vi "#ch_choose.vi"(8 "error in (no error)":errorcluster) -> (0 "error out":errorcluster, 3 "#ch_choise out":enum16{"O2Sim_2ch", "O2Sim_4ch"}(ring))   [LabVIEW 2017, in "ALMA_10201-10401_O2SensorSim System Explorer.lvlib"]
uses:
  ALMA_10201-10401_O2SensorSim System Explorer.lvlib
panel:
  in  "Apply":bool
  in  "#ch_choise":enum16{"O2Sim_2ch", "O2Sim_4ch"}(ring)
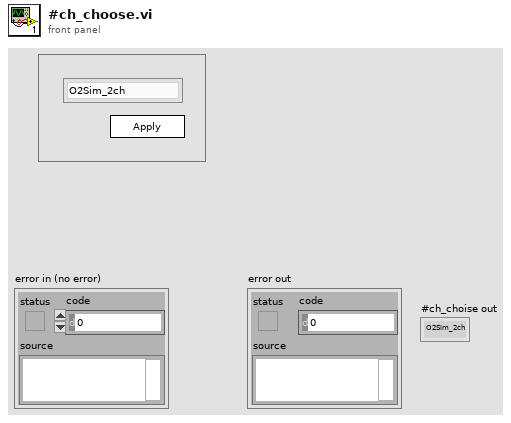
[diagram p1: front panel]
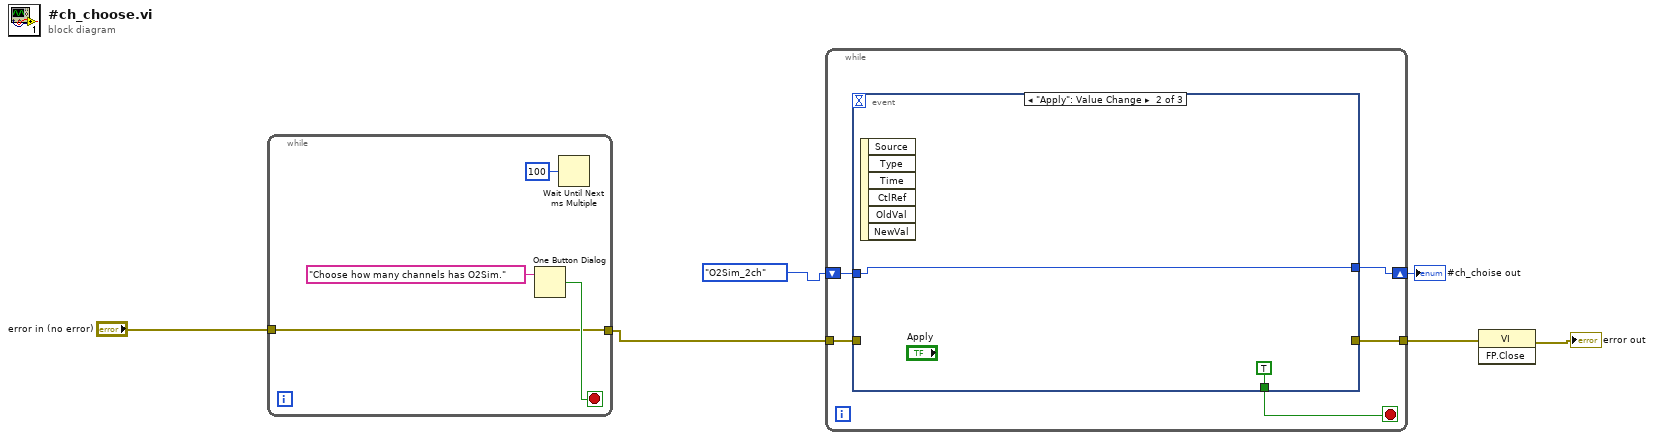
[diagram p0: block diagram]
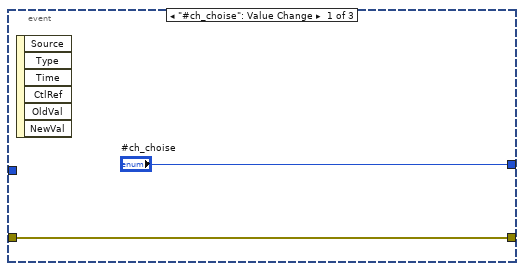
[diagram p2: hidden frame]
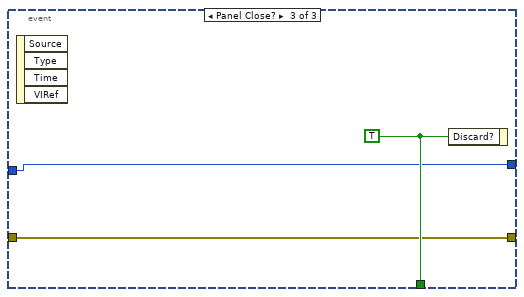
[diagram p3: hidden frame]
diagram:
  n1 = while {
    tunnel: [w7] -> w3
    tunnel: "error in (no error)" -> [w7]
    stop <- w9 stop-if-true
    n2 = One Button Dialog(message="Choose how many channels has O2Sim.") -> (true=w9:bool)  [unwired: 1 in]
    n3 = Wait Until Next ms Multiple(millisecond multiple=u32 100) -> ()  [unwired: 1 out]
  }
  n4 = while {
    tunnel: [w14] -> w6
    tunnel: w3 -> [w13]
    shift-right: [w12] -> w4
    shift-left: enum16{"O2Sim_2ch", "O2Sim_4ch"}."O2Sim_2ch" ("#ch_choise") -> [w11]
    stop <- w15 stop-if-true
    n5 = event shown="[1] \"Apply\": Value Change" {
      selector: _ -> [_ _ _]
      dyn-events: _ -> [_ _ _]
      timeout: _ -> [_ _ _]
      tunnel: [_ TRUE ("Discard?") w22] -> w15
      tunnel: [w17 _ w21] -> w14
      tunnel: w13 -> [w17 _ w21]
      tunnel: ["#ch_choise" w19 w20] -> w12
      tunnel: w11 -> [_ w19 w20]
      event "#ch_choise": Value Change {
        n6 = event-data() -> ()  [unwired: 1 in, 6 out]
      }
      event "Apply": Value Change {
        n7 = event-data() -> ()  [unwired: 1 in, 6 out]
      }
      event Panel Close? {
        w22 = TRUE ("Discard?")
        n8 = event-data() -> ()  [unwired: 1 in, 4 out]
        n9 = event-data("Discard?"=w22) -> ()  [unwired: 1 in, 1 out]
      }
    }
  }
  "#ch_choise out" <- w4
  n10 = invoke class="VI" method="FP.Close"(error in=w6) -> (error out=→"error out":errorcluster)  [unwired: 2 in, 2 out]
